vi "6_Formula loop(170382,170307).vi"() -> ()   [LabVIEW 2015]
panel:
  out "XY Graph":cluster{dbl[], dbl[]}[](graph)=[{[0.0, 0.05, 0.1, 0.15000000000000002, 0.2, 0.25, 0.30000000000000004, 0.35000000000000003, 0.4, 0.45, 0.5, 0.55, 0.6000000000000001, 0.65, 0.7000000000000001, 0.75, 0.8, 0.8500000000000001, 0.9, 0.9500000000000001, 1.0, 1.05, 1.1, 1.1500000000000001, 1.2000000000000002, 1.25, 1.3, 1.35, 1.4000000000000001, 1.4500000000000002, 1.5, 1.55, 1.6, 1.6500000000000001, 1.7000000000000002, 1.75, 1.8, 1.85, 1.9000000000000001, 1.9500000000000002, 2.0, 2.0500000000000003, 2.1, 2.15, 2.2, 2.25, 2.3000000000000003, 2.35, 2.4000000000000004, 2.45, 2.5, 2.5500000000000003, 2.6, 2.6500000000000004, 2.7, 2.75, 2.8000000000000003, 2.85, 2.9000000000000004, 2.95, 3.0, 3.0500000000000003, 3.1, 3.1500000000000004, 3.2, 3.25, 3.3000000000000003, 3.35, 3.4000000000000004, 3.45, 3.5, 3.5500000000000003, 3.6, 3.6500000000000004, 3.7, 3.75, 3.8000000000000003, 3.85, 3.9000000000000004, 3.95, 4.0, 4.05, 4.1000000000000005, 4.15, 4.2, 4.25, 4.3, 4.3500000000000005, 4.4, 4.45, 4.5, 4.55, 4.6000000000000005, 4.65, 4.7, 4.75, 4.800000000000001, 4.8500000000000005, 4.9, 4.95, 5.0, 5.050000000000001, 5.1000000000000005, 5.15, 5.2, 5.25, 5.300000000000001, 5.3500000000000005, 5.4, 5.45, 5.5, 5.550000000000001, 5.6000000000000005, 5.65, 5.7, 5.75, 5.800000000000001, 5.8500000000000005, 5.9, 5.95, 6.0, 6.050000000000001, 6.1000000000000005, 6.15, 6.2, 6.25, 6.300000000000001, 6.3500000000000005, 6.4, 6.45, 6.5, 6.550000000000001, 6.6000000000000005, 6.65, 6.7, 6.75, 6.800000000000001, 6.8500000000000005, 6.9, 6.95, 7.0, 7.050000000000001, 7.1000000000000005, 7.15, 7.2, 7.25, 7.300000000000001, 7.3500000000000005, 7.4, 7.45, 7.5, 7.550000000000001, 7.6000000000000005, 7.65, 7.7, 7.75, 7.800000000000001, 7.8500000000000005, 7.9, 7.95, 8.0, 8.05, 8.1, 8.15, 8.200000000000001, 8.25, 8.3, 8.35, 8.4, 8.450000000000001, 8.5, 8.55, 8.6, 8.65, 8.700000000000001, 8.75, 8.8, 8.85, 8.9, 8.950000000000001, 9.0, 9.05, 9.1, 9.15, 9.200000000000001, 9.25, 9.3, 9.35, 9.4, 9.450000000000001, 9.5, 9.55, 9.600000000000001, 9.65, 9.700000000000001, 9.75, 9.8, 9.850000000000001, 9.9, 9.950000000000001, 10.0], [nan, 0.9995833854135666, 0.9983341664682815, 0.9962542164906615, 0.9933466539753061, 0.9896158370180917, 0.9850673555377986, 0.9797080213012896, 0.9735458557716262, 0.9665900758027338, 0.958851077208406, 0.9503404162375622, 0.9410707889917257, 0.9310560088246762, 0.9203109817681301, 0.9088516800311122, 0.8966951136244035, 0.8838593001650503, 0.870363232919426, 0.8562268471467092, 0.8414709848078965, 0.8261173577085875, 0.8101885091467594, 0.7937077741395835, 0.7766992383060218, 0.759187695484469, 0.7411986041670715, 0.7227580428345622, 0.7038926642774715, 0.6846296489914403, 0.6649966577360363, 0.6450217833479722, 0.6247335019009407, 0.6041606233054053, 0.5833322414426285, 0.562277683927964, 0.5410264615989973, 0.5196082178244864, 0.4980526777302181, 0.4763895974378816, 0.45464871341284085, 0.43285969201628055, 0.41105207935660654, 0.389255251534185, 0.36749836537254094, 0.345810309727965, 0.32421965746813913, 0.3027546182088699, 0.2814429918963127, 0.26031212332020554, 0.23938885764158258, 0.2186994970162418, 0.19826975839287084, 0.1781247325622197, 0.15828884453104805, 0.13878581529175696, 0.11963862505568022, 0.10086947801492785, 0.08249976869447653, 0.06455004995289051, 0.0470400026866224, 0.02998840728932352, 0.013413116913964674, -0.002668967418142559, -0.018241919821118776, -0.03329081062464873, -0.04780172549795413, -0.061761782589074554, -0.07515914765495048, -0.08798304716186357, -0.10022377933989138, -0.11187272317914371, -0.12292234535968123, -0.1333662051111506, -0.1431989570022955, -0.152416351664625, -0.16101523445861032, -0.16899354209484865, -0.17635029722666, -0.18308560103456, -0.18920062382698205, -0.19469759368548026, -0.19957978318644162, -0.20385149423504734, -0.20751804105085433, -0.210585731347902, -0.2130618457556872, -0.214954615530678, -0.21627319861125363, -0.21702765407205366, -0.21722891503668823, -0.21688876011060143, -0.21601978339857922, -0.21463536317395254, -0.2127496292689576, -0.2103774292579743, -0.20753429350746674, -0.20423639916839445, -0.20050053318863928, -0.19634405442461025, -0.1917848549326277, -0.18684132052196162, -0.1815322906524965, -0.17587701776091347, -0.16989512610002944, -0.16360657017649372, -0.1570315928724341, -0.15019068333685145, -0.14310453473259022, -0.13579400192456778, -0.1282800591946167, -0.12058375806779482, -0.112726185334343, -0.10472842135062112, -0.09661149870133992, -0.08839636130421885, -0.08010382403685458, -0.07175453296407844, -0.06336892624241287, -0.054967195776426996, -0.04656924969982098, -0.038194675751965515, -0.02986270561837623, -0.021592180301222234, -0.01340151658346716, -0.005308674647609091, 0.0026688730927540635, 0.010514171893158479, 0.01821081325788963, 0.02574296214960577, 0.03309538278274085, 0.04025346295767621, 0.04720323689596646, 0.05393140654027073, 0.060425361286059444, 0.06667319611564705, 0.07266372810861896, 0.07838651130627908, 0.08383184991133334, 0.08899080980762934, 0.09385522838839844, 0.09841772268507294, 0.10267169579237696, 0.10661134158900856, 0.11023164775682681, 0.11352839710503525, 0.11649816720939243, 0.11913832837998402, 0.12144703997454417, 0.12342324507771418, 0.12506666356996518, 0.1263777836131808, 0.12735785158309032, 0.1280088604818562, 0.1283335368671429, 0.12833532633692596, 0.12801837761212884, 0.12738752526190047, 0.12644827111895848, 0.12520676443492074, 0.12366978082792272, 0.12184470007706825, 0.11973948282038104, 0.11736264621490909, 0.11472323861948444, 0.11183081336234427, 0.10869540165738473, 0.10532748473423532, 0.1017379652486048, 0.09793813804047136, 0.09393966030864591, 0.08975452127105114, 0.08539501138071086, 0.0808736911679385, 0.07620335977956114, 0.07139702328619342, 0.06646786282860928, 0.06142920267413428, 0.0562944782536949, 0.0510772042497379, 0.04579094280463962, 0.04044927191849845, 0.03506575410432441, 0.029653905367610135, 0.024227164576113683, 0.018798863284371196, 0.01338219607602814, 0.00799019148551174, 0.002635683558867847, -0.0026687158882180415, -0.007910644259137822, -0.01307801435777511, -0.018159039710727225, -0.023142258980702993, -0.028016559423808676, -0.03277119934587422, -0.037395829515502896, -0.041880513494121245, -0.04621574684599205, -0.050392475193889334, -0.05440211108893698]}, ...(2 in all)]
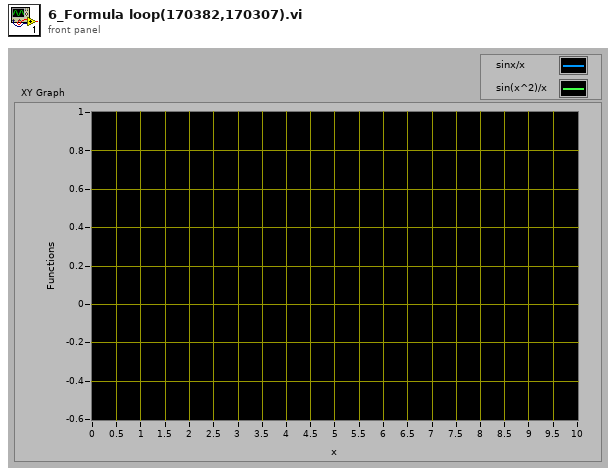
[diagram p1: front panel]
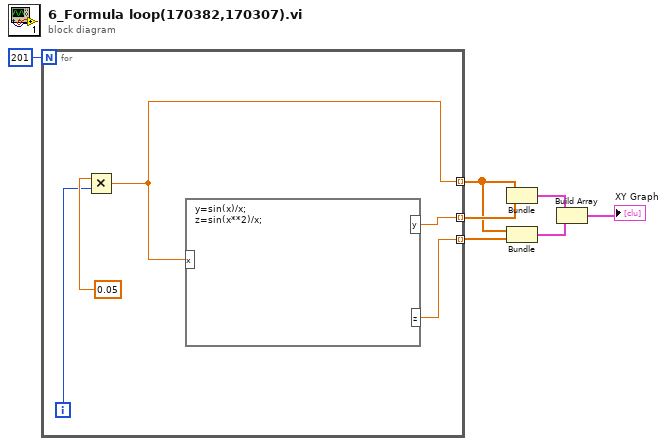
[diagram p0: block diagram]
diagram:
  n1 = for {
    N: 201 -> [_]
    tunnel: [w10] -> w6 mode=indexing
    tunnel: [w8] -> w4 mode=indexing
    tunnel: [w9] -> w5 mode=indexing
    i -> [w11]
    n2 = Multiply(x=0.05, y=w11) -> (x*y=w8:dbl)
    n3 = formula code="y=sin(x)/x;\nz=sin(x**2)/x;"("x"=w8) -> ("y"=w10:dbl, "z"=w9:dbl)
  }
  n4 = Bundle(w4, w6) -> (w2:cluster{dbl[], dbl[]})  [unwired: 1 in]
  n5 = Bundle(w4, w5) -> (w3:cluster{dbl[], dbl[]})  [unwired: 1 in]
  n6 = Build Array(w2, w3) -> (→"XY Graph":cluster{dbl[], dbl[]}[])
